vi "Read String Data.vi"(8 "error in (no error)":errorcluster, 11 "class string in":refnum<class "Parent.lvclass">) -> (0 "error out":errorcluster, 2 "String Data":string, 3 "class string out":refnum<class "Parent.lvclass">)   [LabVIEW 2023, in "Parent.lvclass"]
doc: "This is a member VI of Parent.lvclass, which gets the string data for Parent.ctl, a data member of Parent.lvclass."
uses:
  Parent.lvclass
  Parent.lvclass/Parent.ctl
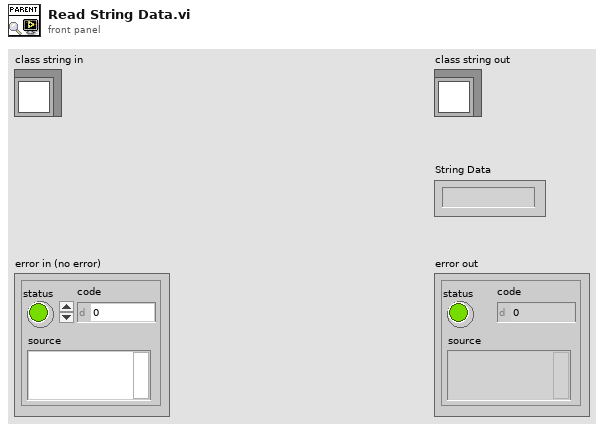
[diagram p1: front panel]
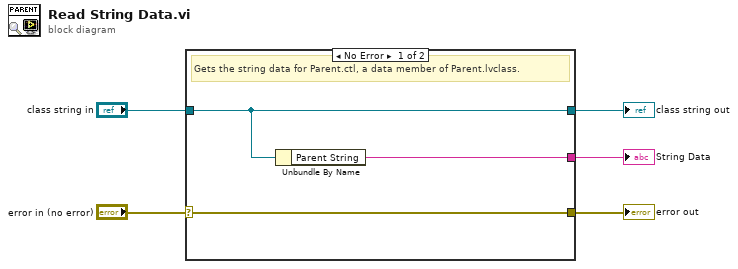
[diagram p0: block diagram]
diagram:
  n1 = case shown="No Error" "error in (no error)" {
    selector: "error in (no error)" -> [w8 w9]
    tunnel: [w8 w9] -> w4
    tunnel: [w7 w10] -> w2
    tunnel: "class string in" -> [w7 w10]
    tunnel: [w6 _] -> w1
    frame No Error {
      # "Gets the string data for Parent.ctl, a data member of Parent.lvclass."
      n2 = Unbundle By Name(w7) -> ("Parent String"=w6:string)
    }
    frame Error {
    }
  }
  "error out" <- w4
  "class string out" <- w2
  "String Data" <- w1
